vi "PH_gentec_P-Link.ProcCases.vi"(0 "i ref in":refnum<vi>, 1 "selector":string, 2 "Data":T1, 3 "call cluster":T2={"Object"="", "Selector"="", "CallType"=enum."synchronous", "Async Object"="", "Async Selector"="", "Data Descriptor"="", "Data"=[], "Error #"=0, "Expire"=0}, 5 "error in":errorcluster) -> (14 "i ref out":refnum<vi>, 17 "answer cluster":T2={"Object"="", "Selector"="", "CallType"=enum."synchronous", "Async Object"="", "Async Selector"="", "Data Descriptor"="", "Data"=[], "Error #"=0, "Expire"=0}, 19 "error out":errorcluster)   [LabVIEW 2014, in "PH_gentec_P-Link.lvlib"]
doc: "This method is called by a process from within the default case in the event loop. The methods of a class that are linked to events will be called from THIS method. Add your code here."
uses:
  PH_gentec_P-Link.lvlib
  CS_Core/CSSystem/CoreDefs/CoreDefs.call_type.ctl
  CS_Core/BaseProcess/BaseProcess.descriptor string definition.ctl
  CS_Core/CSSystem/CoreDefs/CoreDefs.rawDataType.ctl
  instr.lib/Gentec-M-Link/Driver/Type Defs/gentec-M-Link.Measurement Mode.ctl
  instr.lib/Gentec-M-Link/Driver/Type Defs/gentec-M-Link.Trigger Polarity.ctl
  instr.lib/Gentec-M-Link/Driver/Type Defs/gentec-M-Link.Trigger Source.ctl
  CS_Core/CSSystem/CoreLib/CoreLib.string 2 byte array.vi
  CS_Core/CSSystem/CoreLib/CoreLib.byte array 2 short.vi
  CS_Core/CSSystem/CoreLib/CoreLib.byte array 2 int.vi
  CS_Core/CSSystem/CoreLib/CoreLib.lvlib
  CS_Core/BaseProcess/BaseProcess.lvlib
  CS_Core/CAEObj/CAEObj.lvlib
  PH_Basics/PH_PSDBWriter/PH_PSDBWriter.lvlib
  instr.lib/Gentec-M-Link/gentec-M-Link - Driver.lvlib
  PH_Basics/PH_Powermeter_BaseClass/PH_Powermeter_BaseClass.lvlib
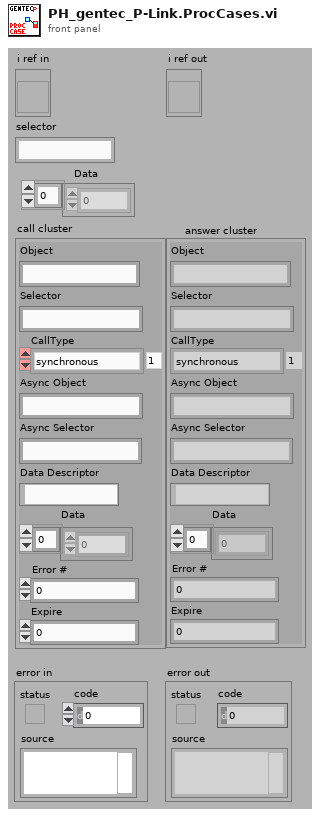
[diagram p1: front panel]
types:
  T1 = typedef "CoreDefs.rawDataType.ctl" = i8[]
  T2 = typedef "CoreDefs.call_type.ctl" = cluster{"Object":string, "Selector":string, "CallType":enum16{"simple", "synchronous", "asynchronous"}, "Async Object":string, "Async Selector":string, "Data Descriptor":T3, "Data":T1, "Error #":i32, "Expire":u32}
  T3 = typedef "BaseProcess.lvlib/BaseProcess.descriptor string definition.ctl" = string
  T4 = typedef "PH_gentec_P-Link.lvlib/PH_gentec_P-Link.i attribute.ctl" = cluster{"GUI References":cluster{"Wanted Head Settings":refnum<vi>, "Current Head Settings":refnum<vi>, "Set Auto Range":refnum<vi>, "Trigger Polarity":refnum<vi>, "Trigger Source":refnum<vi>, "Waveform Averages":refnum<vi>, "Continuous":refnum<vi>, "get one Value":refnum<vi>}, "Wanted Head Settings":T5, "Current Head Settings":T5}
  T5 = typedef "PH_gentec_P-Link.lvlib/PH_gentec_P-Link.Head Settings.ctl" = cluster{"Measurement Mode":T6, "Enable Anticipation":bool, "Set Auto Range":bool, "Block Signal":bool, "Set Head Attenuator":bool, "Enable SSE":bool, "Trigger Polarity":T7, "Trigger Source":T8, "Waveform Averages":T9, "Set Zero":i32, "Current":i32, "Start Data Flow":bool}
  T6 = typedef "gentec-M-Link - Driver.lvlib/gentec-M-Link.Measurement Mode.ctl" = u16
  T7 = typedef "gentec-M-Link - Driver.lvlib/gentec-M-Link.Trigger Polarity.ctl" = u16
  T8 = typedef "gentec-M-Link - Driver.lvlib/gentec-M-Link.Trigger Source.ctl" = u16
  T9 = typedef "gentec-M-Link - Driver.lvlib/gentec-M-Link.Waveform Averages.ctl" = u16
  T10 = typedef "PH_PSDBWriter.lvlib/PH_PSDBWriter.PHELIX-Subsystems.ctl" = i32
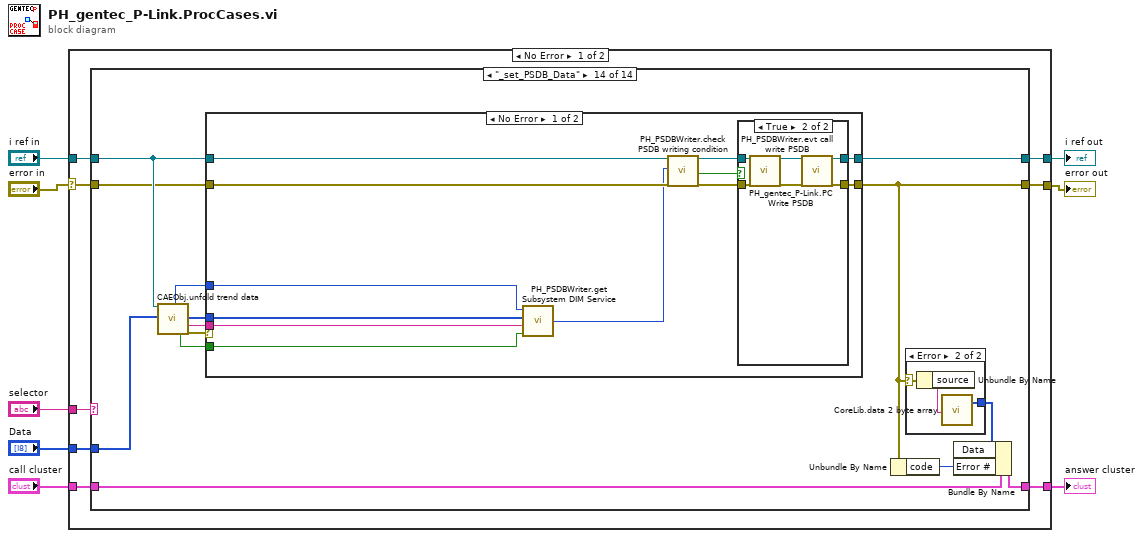
[diagram p0: block diagram]
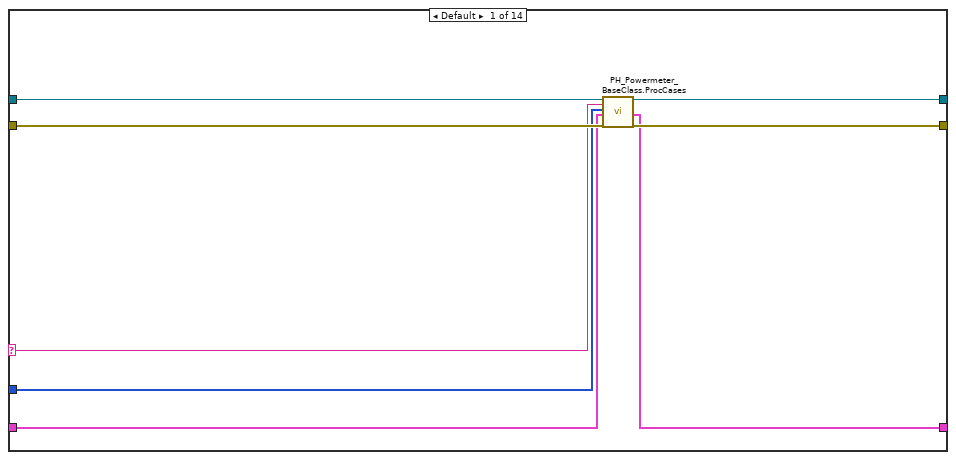
[diagram p2: hidden frame]
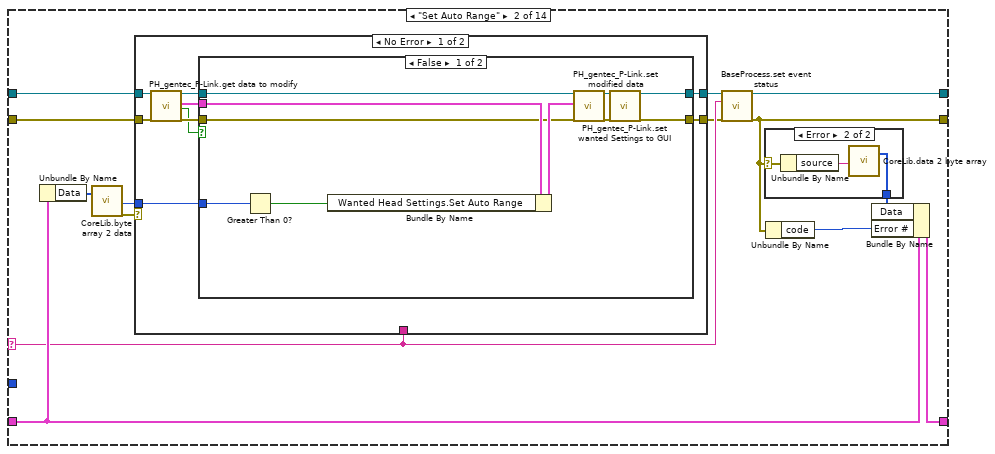
[diagram p3: hidden frame]
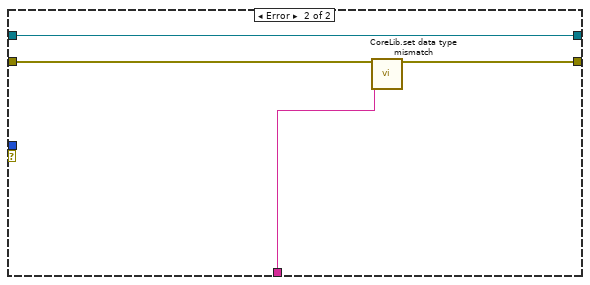
[diagram p6: hidden frame]
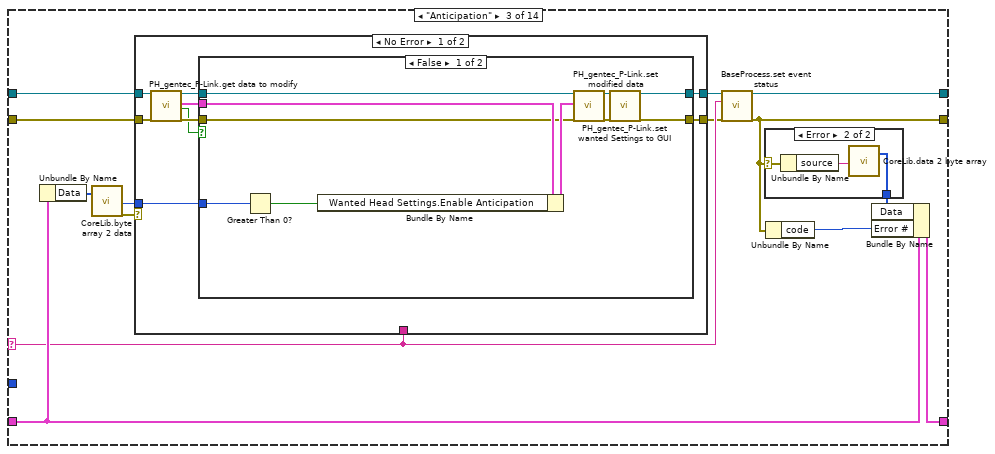
[diagram p7: hidden frame]
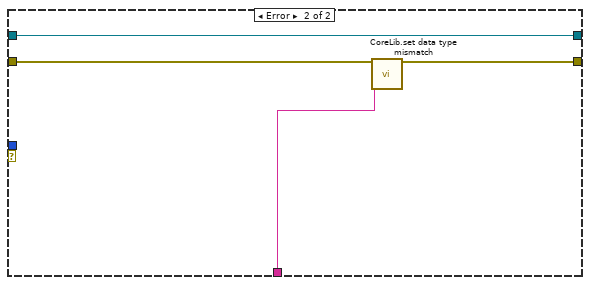
[diagram p10: hidden frame]
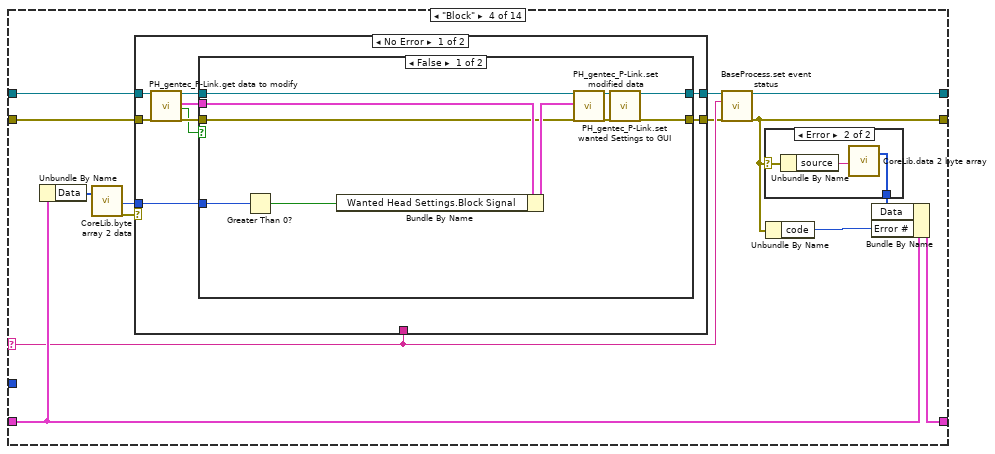
[diagram p11: hidden frame]
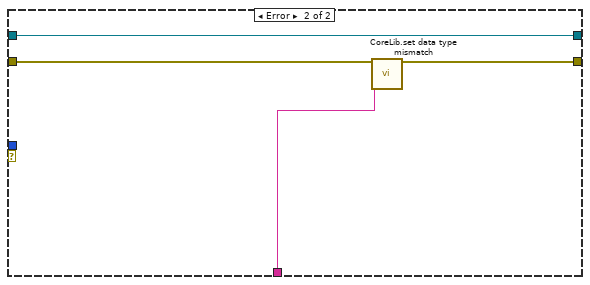
[diagram p14: hidden frame]
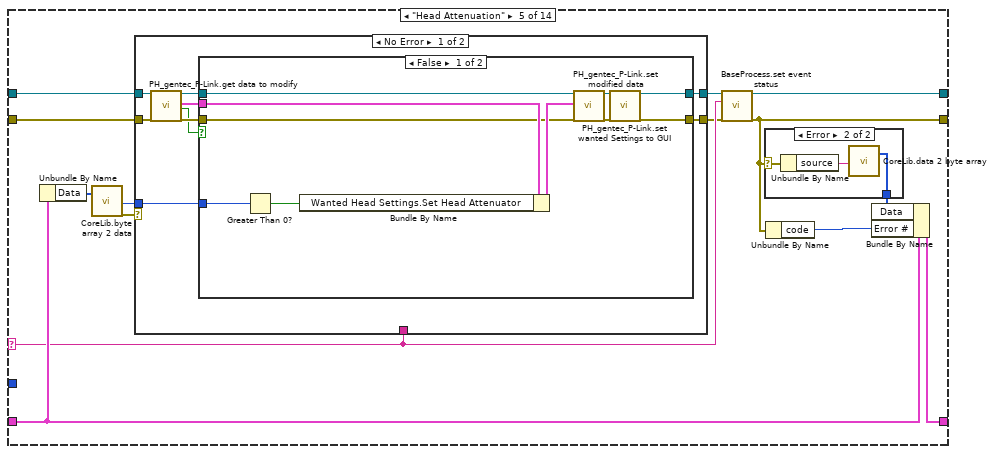
[diagram p15: hidden frame]
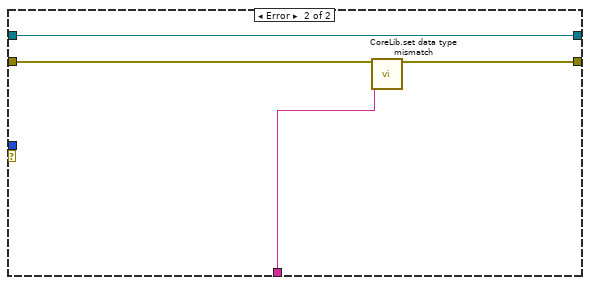
[diagram p18: hidden frame]
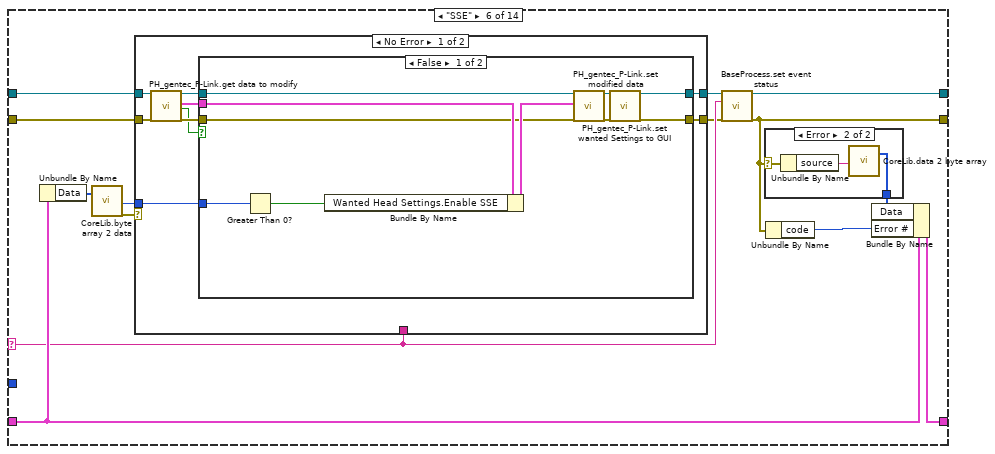
[diagram p19: hidden frame]
diagram:
  n1 = case shown="No Error" "error in" {
    selector: "error in" -> [w9 w553]
    tunnel: "selector" -> [w16 _]
    tunnel: [w15 w552] -> w7
    tunnel: "call cluster" -> [w14 w552]
    tunnel: "i ref in" -> [w13 w554]
    tunnel: [w12 w554] -> w4
    tunnel: [w11 w553] -> w1
    tunnel: "Data" -> [w10 _]
    frame No Error {
      n2 = case shown="\"_set_PSDB_Data\"" w16 {
        selector: w16 -> [w19 w32 w74 w116 w158 w200 w242 w288 w332 w376 w418 w461 w491 _]
        tunnel: w13 -> [w18 w38 w80 w122 w164 w206 w248 w294 w338 w382 w424 w467 w497 w517]
        tunnel: [w24 w33 w75 w117 w159 w201 w243 w289 w333 w377 w419 w462 w492 w516] -> w12
        tunnel: w14 -> [w20 w35 w77 w119 w161 w203 w245 w291 w335 w379 w421 w464 w494 w525]
        tunnel: [w21 w26 w68 w110 w152 w194 w236 w282 w326 w370 w412 w458 w488 w523] -> w15
        tunnel: w9 -> [w23 w37 w79 w121 w163 w205 w247 w293 w337 w381 w423 w466 w496 w514]
        tunnel: [w22 w34 w76 w118 w160 w202 w244 w290 w334 w378 w420 w463 w493 w515] -> w11
        tunnel: w10 -> [w17 _ _ _ _ _ _ _ _ _ _ _ _ w513]
        frame Default {
          # "In the default case, always call the ProcCase method of the parent class"
          n3 = call "PH_Powermeter_BaseClass.ProcCases.vi"("i ref in"=w18, "selector"=w19, "Data"=w17, "call cluster"=w20, "error in"=w23) -> ("i ref out"=w24:refnum<vi>, "answer cluster"=w21:T2, "error out"=w22:errorcluster)  [unwired: 12 in]
        }
        frame "Set Auto Range" {
          n4 = Unbundle By Name(w35) -> ("Data"=w29:T1)
          n5 = call-poly "CoreLib.byte array 2 data.vi"("byteArray"=w29) -> ("i16"=w28:i16, "error out"=w27:errorcluster)  [unwired: 16 in, 1 out]
          n6 = case shown="No Error" w27 {
            tunnel: [w48 w66] -> w30
            tunnel: w38 -> [w50 w66]
            tunnel: w37 -> [w47 w65]
            tunnel: [w45 w64] -> w31
            tunnel: w32 -> [_ w63]
            tunnel: w28 -> [w42 _]
            frame No Error {
              n7 = call "PH_gentec_P-Link.get data to modify.vi"("i ref in"=w50, "error in (no error)"=w47) -> ("i ref out"=w49:refnum<vi>, "i attribute"=w43:T4, "timed out"=w44:bool, "error out"=w46:errorcluster)  [unwired: 14 in]
              n8 = case shown="False" w44 {
                tunnel: w49 -> [w60 w62]
                tunnel: [w52 w62] -> w48
                tunnel: w46 -> [w55 w61]
                tunnel: [w51 w61] -> w45
                tunnel: w43 -> [w57 _]
                tunnel: w42 -> [w56 _]
                frame False {
                  n9 = Greater Than 0?(x=w56) -> (x > 0?=w53:bool)
                  n10 = Bundle By Name(cluster=w57, "Wanted Head Settings.Set Auto Range"=w53) -> (w58:T4)
                  n11 = call "PH_gentec_P-Link.set modified data.vi"("i ref in"=w60, "i attribute"=w58, "error in (no error)"=w55) -> ("i ref out"=w54:refnum<vi>, "error out"=w59:errorcluster)  [unwired: 15 in]
                  n12 = call "PH_gentec_P-Link.set wanted Settings to GUI.vi"("i ref in"=w54, "error in"=w59) -> ("i ref out"=w52:refnum<vi>, "error out"=w51:errorcluster)  [unwired: 16 in]
                }
                frame True {
                }
              }
            }
            frame Error {
              n13 = call "CoreLib.set data type mismatch.vi"("error in (no error)"=w65, "error source"=w63) -> ("error out"=w64:errorcluster)  [unwired: 17 in]
            }
          }
          n14 = call "BaseProcess.set event status.vi"("i ref in"=w30, "EventStatus"=w32, "error in (no error)"=w31) -> ("i ref out"=w33:refnum<vi>, "error out"=w34:errorcluster)  [unwired: 14 in, 1 out]
          n15 = case shown="Error" w34 {
            selector: w34 -> [_ w41]
            tunnel: [_ w39] -> w25
            frame No Error {
            }
            frame Error {
              n16 = Unbundle By Name(w41) -> ("source"=w40:string)
              n17 = call-poly "CoreLib.data 2 byte array.vi"("string"=w40) -> ("byteArray out"=w39:T1)  [unwired: 18 in]
            }
          }
          n18 = Unbundle By Name(w34) -> ("code"=w36:i32)
          n19 = Bundle By Name(cluster=w35, "Data"=w25, "Error #"=w36) -> (w26:T2)
        }
        frame "Anticipation" {
          n20 = Unbundle By Name(w77) -> ("Data"=w71:T1)
          n21 = call-poly "CoreLib.byte array 2 data.vi"("byteArray"=w71) -> ("i16"=w70:i16, "error out"=w69:errorcluster)  [unwired: 16 in, 1 out]
          n22 = case shown="No Error" w69 {
            tunnel: [w90 w108] -> w72
            tunnel: w80 -> [w92 w108]
            tunnel: w79 -> [w89 w107]
            tunnel: [w87 w106] -> w73
            tunnel: w74 -> [_ w105]
            tunnel: w70 -> [w84 _]
            frame No Error {
              n23 = call "PH_gentec_P-Link.get data to modify.vi"("i ref in"=w92, "error in (no error)"=w89) -> ("i ref out"=w91:refnum<vi>, "i attribute"=w85:T4, "timed out"=w86:bool, "error out"=w88:errorcluster)  [unwired: 14 in]
              n24 = case shown="False" w86 {
                tunnel: w91 -> [w102 w104]
                tunnel: [w94 w104] -> w90
                tunnel: w88 -> [w97 w103]
                tunnel: [w93 w103] -> w87
                tunnel: w85 -> [w99 _]
                tunnel: w84 -> [w98 _]
                frame False {
                  n25 = Greater Than 0?(x=w98) -> (x > 0?=w95:bool)
                  n26 = Bundle By Name(cluster=w99, "Wanted Head Settings.Enable Anticipation"=w95) -> (w100:T4)
                  n27 = call "PH_gentec_P-Link.set modified data.vi"("i ref in"=w102, "i attribute"=w100, "error in (no error)"=w97) -> ("i ref out"=w96:refnum<vi>, "error out"=w101:errorcluster)  [unwired: 15 in]
                  n28 = call "PH_gentec_P-Link.set wanted Settings to GUI.vi"("i ref in"=w96, "error in"=w101) -> ("i ref out"=w94:refnum<vi>, "error out"=w93:errorcluster)  [unwired: 16 in]
                }
                frame True {
                }
              }
            }
            frame Error {
              n29 = call "CoreLib.set data type mismatch.vi"("error in (no error)"=w107, "error source"=w105) -> ("error out"=w106:errorcluster)  [unwired: 17 in]
            }
          }
          n30 = call "BaseProcess.set event status.vi"("i ref in"=w72, "EventStatus"=w74, "error in (no error)"=w73) -> ("i ref out"=w75:refnum<vi>, "error out"=w76:errorcluster)  [unwired: 14 in, 1 out]
          n31 = case shown="Error" w76 {
            selector: w76 -> [_ w83]
            tunnel: [_ w81] -> w67
            frame No Error {
            }
            frame Error {
              n32 = Unbundle By Name(w83) -> ("source"=w82:string)
              n33 = call-poly "CoreLib.data 2 byte array.vi"("string"=w82) -> ("byteArray out"=w81:T1)  [unwired: 18 in]
            }
          }
          n34 = Unbundle By Name(w76) -> ("code"=w78:i32)
          n35 = Bundle By Name(cluster=w77, "Data"=w67, "Error #"=w78) -> (w68:T2)
        }
        frame "Block" {
          n36 = Unbundle By Name(w119) -> ("Data"=w113:T1)
          n37 = call-poly "CoreLib.byte array 2 data.vi"("byteArray"=w113) -> ("i16"=w112:i16, "error out"=w111:errorcluster)  [unwired: 16 in, 1 out]
          n38 = case shown="No Error" w111 {
            tunnel: [w132 w150] -> w114
            tunnel: w122 -> [w134 w150]
            tunnel: w121 -> [w131 w149]
            tunnel: [w129 w148] -> w115
            tunnel: w116 -> [_ w147]
            tunnel: w112 -> [w126 _]
            frame No Error {
              n39 = call "PH_gentec_P-Link.get data to modify.vi"("i ref in"=w134, "error in (no error)"=w131) -> ("i ref out"=w133:refnum<vi>, "i attribute"=w127:T4, "timed out"=w128:bool, "error out"=w130:errorcluster)  [unwired: 14 in]
              n40 = case shown="False" w128 {
                tunnel: w133 -> [w144 w146]
                tunnel: [w136 w146] -> w132
                tunnel: w130 -> [w139 w145]
                tunnel: [w135 w145] -> w129
                tunnel: w127 -> [w141 _]
                tunnel: w126 -> [w140 _]
                frame False {
                  n41 = Greater Than 0?(x=w140) -> (x > 0?=w137:bool)
                  n42 = Bundle By Name(cluster=w141, "Wanted Head Settings.Block Signal"=w137) -> (w142:T4)
                  n43 = call "PH_gentec_P-Link.set modified data.vi"("i ref in"=w144, "i attribute"=w142, "error in (no error)"=w139) -> ("i ref out"=w138:refnum<vi>, "error out"=w143:errorcluster)  [unwired: 15 in]
                  n44 = call "PH_gentec_P-Link.set wanted Settings to GUI.vi"("i ref in"=w138, "error in"=w143) -> ("i ref out"=w136:refnum<vi>, "error out"=w135:errorcluster)  [unwired: 16 in]
                }
                frame True {
                }
              }
            }
            frame Error {
              n45 = call "CoreLib.set data type mismatch.vi"("error in (no error)"=w149, "error source"=w147) -> ("error out"=w148:errorcluster)  [unwired: 17 in]
            }
          }
          n46 = call "BaseProcess.set event status.vi"("i ref in"=w114, "EventStatus"=w116, "error in (no error)"=w115) -> ("i ref out"=w117:refnum<vi>, "error out"=w118:errorcluster)  [unwired: 14 in, 1 out]
          n47 = case shown="Error" w118 {
            selector: w118 -> [_ w125]
            tunnel: [_ w123] -> w109
            frame No Error {
            }
            frame Error {
              n48 = Unbundle By Name(w125) -> ("source"=w124:string)
              n49 = call-poly "CoreLib.data 2 byte array.vi"("string"=w124) -> ("byteArray out"=w123:T1)  [unwired: 18 in]
            }
          }
          n50 = Unbundle By Name(w118) -> ("code"=w120:i32)
          n51 = Bundle By Name(cluster=w119, "Data"=w109, "Error #"=w120) -> (w110:T2)
        }
        frame "Head Attenuation" {
          n52 = Unbundle By Name(w161) -> ("Data"=w155:T1)
          n53 = call-poly "CoreLib.byte array 2 data.vi"("byteArray"=w155) -> ("i16"=w154:i16, "error out"=w153:errorcluster)  [unwired: 16 in, 1 out]
          n54 = case shown="No Error" w153 {
            tunnel: [w174 w192] -> w156
            tunnel: w164 -> [w176 w192]
            tunnel: w163 -> [w173 w191]
            tunnel: [w171 w190] -> w157
            tunnel: w158 -> [_ w189]
            tunnel: w154 -> [w168 _]
            frame No Error {
              n55 = call "PH_gentec_P-Link.get data to modify.vi"("i ref in"=w176, "error in (no error)"=w173) -> ("i ref out"=w175:refnum<vi>, "i attribute"=w169:T4, "timed out"=w170:bool, "error out"=w172:errorcluster)  [unwired: 14 in]
              n56 = case shown="False" w170 {
                tunnel: w175 -> [w186 w188]
                tunnel: [w178 w188] -> w174
                tunnel: w172 -> [w181 w187]
                tunnel: [w177 w187] -> w171
                tunnel: w169 -> [w183 _]
                tunnel: w168 -> [w182 _]
                frame False {
                  n57 = Greater Than 0?(x=w182) -> (x > 0?=w179:bool)
                  n58 = Bundle By Name(cluster=w183, "Wanted Head Settings.Set Head Attenuator"=w179) -> (w184:T4)
                  n59 = call "PH_gentec_P-Link.set modified data.vi"("i ref in"=w186, "i attribute"=w184, "error in (no error)"=w181) -> ("i ref out"=w180:refnum<vi>, "error out"=w185:errorcluster)  [unwired: 15 in]
                  n60 = call "PH_gentec_P-Link.set wanted Settings to GUI.vi"("i ref in"=w180, "error in"=w185) -> ("i ref out"=w178:refnum<vi>, "error out"=w177:errorcluster)  [unwired: 16 in]
                }
                frame True {
                }
              }
            }
            frame Error {
              n61 = call "CoreLib.set data type mismatch.vi"("error in (no error)"=w191, "error source"=w189) -> ("error out"=w190:errorcluster)  [unwired: 17 in]
            }
          }
          n62 = call "BaseProcess.set event status.vi"("i ref in"=w156, "EventStatus"=w158, "error in (no error)"=w157) -> ("i ref out"=w159:refnum<vi>, "error out"=w160:errorcluster)  [unwired: 14 in, 1 out]
          n63 = case shown="Error" w160 {
            selector: w160 -> [_ w167]
            tunnel: [_ w165] -> w151
            frame No Error {
            }
            frame Error {
              n64 = Unbundle By Name(w167) -> ("source"=w166:string)
              n65 = call-poly "CoreLib.data 2 byte array.vi"("string"=w166) -> ("byteArray out"=w165:T1)  [unwired: 18 in]
            }
          }
          n66 = Unbundle By Name(w160) -> ("code"=w162:i32)
          n67 = Bundle By Name(cluster=w161, "Data"=w151, "Error #"=w162) -> (w152:T2)
        }
        frame "SSE" {
          n68 = Unbundle By Name(w203) -> ("Data"=w197:T1)
          n69 = call-poly "CoreLib.byte array 2 data.vi"("byteArray"=w197) -> ("i16"=w196:i16, "error out"=w195:errorcluster)  [unwired: 16 in, 1 out]
          n70 = case shown="No Error" w195 {
            tunnel: [w216 w234] -> w198
            tunnel: w206 -> [w218 w234]
            tunnel: w205 -> [w215 w233]
            tunnel: [w213 w232] -> w199
            tunnel: w200 -> [_ w231]
            tunnel: w196 -> [w210 _]
            frame No Error {
              n71 = call "PH_gentec_P-Link.get data to modify.vi"("i ref in"=w218, "error in (no error)"=w215) -> ("i ref out"=w217:refnum<vi>, "i attribute"=w211:T4, "timed out"=w212:bool, "error out"=w214:errorcluster)  [unwired: 14 in]
              n72 = case shown="False" w212 {
                tunnel: w217 -> [w228 w230]
                tunnel: [w220 w230] -> w216
                tunnel: w214 -> [w223 w229]
                tunnel: [w219 w229] -> w213
                tunnel: w211 -> [w225 _]
                tunnel: w210 -> [w224 _]
                frame False {
                  n73 = Greater Than 0?(x=w224) -> (x > 0?=w221:bool)
                  n74 = Bundle By Name(cluster=w225, "Wanted Head Settings.Enable SSE"=w221) -> (w226:T4)
                  n75 = call "PH_gentec_P-Link.set modified data.vi"("i ref in"=w228, "i attribute"=w226, "error in (no error)"=w223) -> ("i ref out"=w222:refnum<vi>, "error out"=w227:errorcluster)  [unwired: 15 in]
                  n76 = call "PH_gentec_P-Link.set wanted Settings to GUI.vi"("i ref in"=w222, "error in"=w227) -> ("i ref out"=w220:refnum<vi>, "error out"=w219:errorcluster)  [unwired: 16 in]
                }
                frame True {
                }
              }
            }
            frame Error {
              n77 = call "CoreLib.set data type mismatch.vi"("error in (no error)"=w233, "error source"=w231) -> ("error out"=w232:errorcluster)  [unwired: 17 in]
            }
          }
          n78 = call "BaseProcess.set event status.vi"("i ref in"=w198, "EventStatus"=w200, "error in (no error)"=w199) -> ("i ref out"=w201:refnum<vi>, "error out"=w202:errorcluster)  [unwired: 14 in, 1 out]
          n79 = case shown="Error" w202 {
            selector: w202 -> [_ w209]
            tunnel: [_ w207] -> w193
            frame No Error {
            }
            frame Error {
              n80 = Unbundle By Name(w209) -> ("source"=w208:string)
              n81 = call-poly "CoreLib.data 2 byte array.vi"("string"=w208) -> ("byteArray out"=w207:T1)  [unwired: 18 in]
            }
          }
          n82 = Unbundle By Name(w202) -> ("code"=w204:i32)
          n83 = Bundle By Name(cluster=w203, "Data"=w193, "Error #"=w204) -> (w194:T2)
        }
        frame "Measurement Mode" {
          n84 = Unbundle By Name(w245) -> ("Data"=w239:T1)
          n85 = call-poly "CoreLib.byte array 2 data.vi"("byteArray"=w239) -> ("i32"=w238:i32, "error out"=w237:errorcluster)  [unwired: 16 in, 1 out]
          n86 = case shown="No Error" w237 {
            tunnel: [w258 w280] -> w240
            tunnel: w248 -> [w260 w280]
            tunnel: w247 -> [w257 w279]
            tunnel: [w255 w278] -> w241
            tunnel: w242 -> [_ w277]
            tunnel: w238 -> [w252 _]
            frame No Error {
              n87 = call "PH_gentec_P-Link.get data to modify.vi"("i ref in"=w260, "error in (no error)"=w257) -> ("i ref out"=w259:refnum<vi>, "i attribute"=w253:T4, "timed out"=w254:bool, "error out"=w256:errorcluster)  [unwired: 14 in]
              n88 = case shown="False" w254 {
                tunnel: w259 -> [w274 w276]
                tunnel: [w262 w276] -> w258
                tunnel: w256 -> [w271 w275]
                tunnel: [w261 w275] -> w255
                tunnel: w253 -> [w269 _]
                tunnel: w252 -> [w268 _]
                frame False {
                  w264 = T6 1 items=["other Mode", "Energymode"] ("Wanted Head Settings.Measurement Mode")
                  w265 = T6 0 items=["other Mode", "Energymode"] ("Wanted Head Settings.Measurement Mode")
                  n89 = Equal?(x=w268, y=1) -> (x = y?=w266:bool)
                  n90 = Select(t=w264, s=w266, f=w265) -> (s? t:f=w263:T6)
                  n91 = Bundle By Name(cluster=w269, "Wanted Head Settings.Measurement Mode"=w263) -> (w272:T4)
                  n92 = call "PH_gentec_P-Link.set modified data.vi"("i ref in"=w274, "i attribute"=w272, "error in (no error)"=w271) -> ("i ref out"=w270:refnum<vi>, "error out"=w273:errorcluster)  [unwired: 15 in]
                  n93 = call "PH_gentec_P-Link.set wanted Settings to GUI.vi"("i ref in"=w270, "error in"=w273) -> ("i ref out"=w262:refnum<vi>, "error out"=w261:errorcluster)  [unwired: 16 in]
                }
                frame True {
                }
              }
            }
            frame Error {
              n94 = call "CoreLib.set data type mismatch.vi"("error in (no error)"=w279, "error source"=w277) -> ("error out"=w278:errorcluster)  [unwired: 17 in]
            }
          }
          n95 = call "BaseProcess.set event status.vi"("i ref in"=w240, "EventStatus"=w242, "error in (no error)"=w241) -> ("i ref out"=w243:refnum<vi>, "error out"=w244:errorcluster)  [unwired: 14 in, 1 out]
          n96 = case shown="Error" w244 {
            selector: w244 -> [_ w251]
            tunnel: [_ w249] -> w235
            frame No Error {
            }
            frame Error {
              n97 = Unbundle By Name(w251) -> ("source"=w250:string)
              n98 = call-poly "CoreLib.data 2 byte array.vi"("string"=w250) -> ("byteArray out"=w249:T1)  [unwired: 18 in]
            }
          }
          n99 = Unbundle By Name(w244) -> ("code"=w246:i32)
          n100 = Bundle By Name(cluster=w245, "Data"=w235, "Error #"=w246) -> (w236:T2)
        }
        frame "Set Trigger Polarity" {
          n101 = Unbundle By Name(w291) -> ("Data"=w285:T1)
          n102 = call-poly "CoreLib.byte array 2 data.vi"("byteArray"=w285) -> ("i32"=w284:i32, "error out"=w283:errorcluster)  [unwired: 16 in, 1 out]
          n103 = case shown="No Error" w283 {
            tunnel: [w304 w324] -> w286
            tunnel: w294 -> [w306 w324]
            tunnel: w293 -> [w303 w323]
            tunnel: [w301 w322] -> w287
            tunnel: w288 -> [_ w321]
            tunnel: w284 -> [w298 _]
            frame No Error {
              n104 = call "PH_gentec_P-Link.get data to modify.vi"("i ref in"=w306, "error in (no error)"=w303) -> ("i ref out"=w305:refnum<vi>, "i attribute"=w299:T4, "timed out"=w300:bool, "error out"=w302:errorcluster)  [unwired: 14 in]
              n105 = case shown="False" w300 {
                tunnel: w305 -> [w316 w320]
                tunnel: [w308 w320] -> w304
                tunnel: w302 -> [w313 w319]
                tunnel: [w307 w319] -> w301
                tunnel: w299 -> [w311 _]
                tunnel: w298 -> [w309 _]
                frame False {
                  n106 = case shown="Default" w309 {
                    tunnel: [w317 w318] -> w310
                    frame 1 {
                      w317 = T7 1 items=["Rising Edge", "Falling Edge"] ("Wanted Head Settings.Trigger Polarity")
                    }
                    frame Default {
                      w318 = T7 0 items=["Rising Edge", "Falling Edge"] ("Wanted Head Settings.Trigger Polarity")
                    }
                  }
                  n107 = Bundle By Name(cluster=w311, "Wanted Head Settings.Trigger Polarity"=w310) -> (w314:T4)
                  n108 = call "PH_gentec_P-Link.set modified data.vi"("i ref in"=w316, "i attribute"=w314, "error in (no error)"=w313) -> ("i ref out"=w312:refnum<vi>, "error out"=w315:errorcluster)  [unwired: 15 in]
                  n109 = call "PH_gentec_P-Link.set wanted Settings to GUI.vi"("i ref in"=w312, "error in"=w315) -> ("i ref out"=w308:refnum<vi>, "error out"=w307:errorcluster)  [unwired: 16 in]
                }
                frame True {
                }
              }
            }
            frame Error {
              n110 = call "CoreLib.set data type mismatch.vi"("error in (no error)"=w323, "error source"=w321) -> ("error out"=w322:errorcluster)  [unwired: 17 in]
            }
          }
          n111 = call "BaseProcess.set event status.vi"("i ref in"=w286, "EventStatus"=w288, "error in (no error)"=w287) -> ("i ref out"=w289:refnum<vi>, "error out"=w290:errorcluster)  [unwired: 14 in, 1 out]
          n112 = case shown="Error" w290 {
            selector: w290 -> [_ w297]
            tunnel: [_ w295] -> w281
            frame No Error {
            }
            frame Error {
              n113 = Unbundle By Name(w297) -> ("source"=w296:string)
              n114 = call-poly "CoreLib.data 2 byte array.vi"("string"=w296) -> ("byteArray out"=w295:T1)  [unwired: 18 in]
            }
          }
          n115 = Unbundle By Name(w290) -> ("code"=w292:i32)
          n116 = Bundle By Name(cluster=w291, "Data"=w281, "Error #"=w292) -> (w282:T2)
        }
        frame "Set Trigger Source" {
          n117 = Unbundle By Name(w335) -> ("Data"=w329:T1)
          n118 = call-poly "CoreLib.byte array 2 data.vi"("byteArray"=w329) -> ("i32"=w328:i32, "error out"=w327:errorcluster)  [unwired: 16 in, 1 out]
          n119 = case shown="No Error" w327 {
            tunnel: [w348 w368] -> w330
            tunnel: w338 -> [w350 w368]
            tunnel: w337 -> [w347 w367]
            tunnel: [w345 w366] -> w331
            tunnel: w332 -> [_ w365]
            tunnel: w328 -> [w342 _]
            frame No Error {
              n120 = call "PH_gentec_P-Link.get data to modify.vi"("i ref in"=w350, "error in (no error)"=w347) -> ("i ref out"=w349:refnum<vi>, "i attribute"=w343:T4, "timed out"=w344:bool, "error out"=w346:errorcluster)  [unwired: 14 in]
              n121 = case shown="False" w344 {
                tunnel: w349 -> [w360 w364]
                tunnel: [w352 w364] -> w348
                tunnel: w346 -> [w357 w363]
                tunnel: [w351 w363] -> w345
                tunnel: w343 -> [w355 _]
                tunnel: w342 -> [w354 _]
                frame False {
                  n122 = case shown="0" w354 {
                    tunnel: [w361 w362] -> w353
                    frame 0 {
                      w361 = T8 0 items=["Internal", "External"] ("Wanted Head Settings.Trigger Source")
                    }
                    frame Default {
                      w362 = T8 1 items=["Internal", "External"] ("Wanted Head Settings.Trigger Source")
                    }
                  }
                  n123 = Bundle By Name(cluster=w355, "Wanted Head Settings.Trigger Source"=w353) -> (w358:T4)
                  n124 = call "PH_gentec_P-Link.set modified data.vi"("i ref in"=w360, "i attribute"=w358, "error in (no error)"=w357) -> ("i ref out"=w356:refnum<vi>, "error out"=w359:errorcluster)  [unwired: 15 in]
                  n125 = call "PH_gentec_P-Link.set wanted Settings to GUI.vi"("i ref in"=w356, "error in"=w359) -> ("i ref out"=w352:refnum<vi>, "error out"=w351:errorcluster)  [unwired: 16 in]
                }
                frame True {
                }
              }
            }
            frame Error {
              n126 = call "CoreLib.set data type mismatch.vi"("error in (no error)"=w367, "error source"=w365) -> ("error out"=w366:errorcluster)  [unwired: 17 in]
            }
          }
          n127 = call "BaseProcess.set event status.vi"("i ref in"=w330, "EventStatus"=w332, "error in (no error)"=w331) -> ("i ref out"=w333:refnum<vi>, "error out"=w334:errorcluster)  [unwired: 14 in, 1 out]
          n128 = case shown="Error" w334 {
            selector: w334 -> [_ w341]
            tunnel: [_ w339] -> w325
            frame No Error {
            }
            frame Error {
              n129 = Unbundle By Name(w341) -> ("source"=w340:string)
              n130 = call-poly "CoreLib.data 2 byte array.vi"("string"=w340) -> ("byteArray out"=w339:T1)  [unwired: 18 in]
            }
          }
          n131 = Unbundle By Name(w334) -> ("code"=w336:i32)
          n132 = Bundle By Name(cluster=w335, "Data"=w325, "Error #"=w336) -> (w326:T2)
        }
        frame "Set Waveform Averages" {
          n133 = Unbundle By Name(w379) -> ("Data"=w373:T1)
          n134 = call-poly "CoreLib.byte array 2 data.vi"("byteArray"=w373) -> ("i32"=w372:i32, "error out"=w371:errorcluster)  [unwired: 16 in, 1 out]
          n135 = case shown="No Error" w371 {
            tunnel: [w392 w410] -> w374
            tunnel: w382 -> [w394 w410]
            tunnel: w381 -> [w391 w409]
            tunnel: [w389 w408] -> w375
            tunnel: w376 -> [_ w407]
            tunnel: w372 -> [w386 _]
            frame No Error {
              n136 = call "PH_gentec_P-Link.get data to modify.vi"("i ref in"=w394, "error in (no error)"=w391) -> ("i ref out"=w393:refnum<vi>, "i attribute"=w387:T4, "timed out"=w388:bool, "error out"=w390:errorcluster)  [unwired: 14 in]
              n137 = case shown="False" w388 {
                tunnel: w393 -> [w404 w406]
                tunnel: [w396 w406] -> w392
                tunnel: w390 -> [w401 w405]
                tunnel: [w395 w405] -> w389
                tunnel: w387 -> [w399 _]
                tunnel: w386 -> [w398 _]
                frame False {
                  n138 = To Unsigned Word Integer(number=w398) -> (unsigned 16bit integer=w397:u16)
                  n139 = Bundle By Name(cluster=w399, "Wanted Head Settings.Waveform Averages"=w397) -> (w402:T4)
                  n140 = call "PH_gentec_P-Link.set modified data.vi"("i ref in"=w404, "i attribute"=w402, "error in (no error)"=w401) -> ("i ref out"=w400:refnum<vi>, "error out"=w403:errorcluster)  [unwired: 15 in]
                  n141 = call "PH_gentec_P-Link.set wanted Settings to GUI.vi"("i ref in"=w400, "error in"=w403) -> ("i ref out"=w396:refnum<vi>, "error out"=w395:errorcluster)  [unwired: 16 in]
                }
                frame True {
                }
              }
            }
            frame Error {
              n142 = call "CoreLib.set data type mismatch.vi"("error in (no error)"=w409, "error source"=w407) -> ("error out"=w408:errorcluster)  [unwired: 17 in]
            }
          }
          n143 = call "BaseProcess.set event status.vi"("i ref in"=w374, "EventStatus"=w376, "error in (no error)"=w375) -> ("i ref out"=w377:refnum<vi>, "error out"=w378:errorcluster)  [unwired: 14 in, 1 out]
          n144 = case shown="Error" w378 {
            selector: w378 -> [_ w385]
            tunnel: [_ w383] -> w369
            frame No Error {
            }
            frame Error {
              n145 = Unbundle By Name(w385) -> ("source"=w384:string)
              n146 = call-poly "CoreLib.data 2 byte array.vi"("string"=w384) -> ("byteArray out"=w383:T1)  [unwired: 18 in]
            }
          }
          n147 = Unbundle By Name(w378) -> ("code"=w380:i32)
          n148 = Bundle By Name(cluster=w379, "Data"=w369, "Error #"=w380) -> (w370:T2)
        }
        frame "Continuous Measurement" {
          n149 = Unbundle By Name(w421) -> ("Data"=w415:T1)
          n150 = call-poly "CoreLib.byte array 2 data.vi"("byteArray"=w415) -> ("i16"=w414:i16, "error out"=w413:errorcluster)  [unwired: 16 in, 1 out]
          n151 = case shown="No Error" w413 {
            tunnel: [w434 w452] -> w416
            tunnel: w424 -> [w436 w452]
            tunnel: w423 -> [w433 w451]
            tunnel: [w431 w450] -> w417
            tunnel: w418 -> [_ w449]
            tunnel: w414 -> [w428 _]
            frame No Error {
              n152 = call "PH_gentec_P-Link.get data to modify.vi"("i ref in"=w436, "error in (no error)"=w433) -> ("i ref out"=w435:refnum<vi>, "i attribute"=w429:T4, "timed out"=w430:bool, "error out"=w432:errorcluster)  [unwired: 14 in]
              n153 = case shown="False" w430 {
                tunnel: w435 -> [w446 w448]
                tunnel: [w438 w448] -> w434
                tunnel: w432 -> [w441 w447]
                tunnel: [w437 w447] -> w431
                tunnel: w429 -> [w443 _]
                tunnel: w428 -> [w442 _]
                frame False {
                  n154 = Greater Than 0?(x=w442) -> (x > 0?=w439:bool)
                  n155 = Bundle By Name(cluster=w443, "Wanted Head Settings.Start Data Flow"=w439) -> (w444:T4)
                  n156 = call "PH_gentec_P-Link.set modified data.vi"("i ref in"=w446, "i attribute"=w444, "error in (no error)"=w441) -> ("i ref out"=w440:refnum<vi>, "error out"=w445:errorcluster)  [unwired: 15 in]
                  n157 = call "PH_gentec_P-Link.set wanted Settings to GUI.vi"("i ref in"=w440, "error in"=w445) -> ("i ref out"=w438:refnum<vi>, "error out"=w437:errorcluster)  [unwired: 16 in]
                }
                frame True {
                }
              }
            }
            frame Error {
              n158 = call "CoreLib.set data type mismatch.vi"("error in (no error)"=w451, "error source"=w449) -> ("error out"=w450:errorcluster)  [unwired: 17 in]
            }
          }
          n159 = call "BaseProcess.set event status.vi"("i ref in"=w416, "EventStatus"=w418, "error in (no error)"=w417) -> ("i ref out"=w419:refnum<vi>, "error out"=w420:errorcluster)  [unwired: 14 in, 1 out]
          n160 = case shown="Error" w420 {
            selector: w420 -> [_ w427]
            tunnel: [_ w425] -> w411
            frame No Error {
            }
            frame Error {
              n161 = Unbundle By Name(w427) -> ("source"=w426:string)
              n162 = call-poly "CoreLib.data 2 byte array.vi"("string"=w426) -> ("byteArray out"=w425:T1)  [unwired: 18 in]
            }
          }
          n163 = Unbundle By Name(w420) -> ("code"=w422:i32)
          n164 = Bundle By Name(cluster=w421, "Data"=w411, "Error #"=w422) -> (w412:T2)
        }
        frame "Current Measurement" {
          n165 = call "PH_gentec_P-Link.get data to modify.vi"("i ref in"=w467, "error in (no error)"=w466) -> ("i ref out"=w456:refnum<vi>, "i attribute"=w453:T4, "timed out"=w454:bool, "error out"=w455:errorcluster)  [unwired: 14 in]
          n166 = case shown="False" w454 {
            tunnel: w456 -> [w477 w479]
            tunnel: [w469 w479] -> w459
            tunnel: w455 -> [w474 w478]
            tunnel: [w468 w478] -> w460
            tunnel: w453 -> [w472 _]
            frame False {
              n167 = Unbundle By Name(w472) -> ("Wanted Head Settings.Current"=w471:i32)
              n168 = Increment(x=w471) -> (x+1=w470:i32)
              n169 = Bundle By Name(cluster=w472, "Wanted Head Settings.Current"=w470) -> (w475:T4)
              n170 = call "PH_gentec_P-Link.set modified data.vi"("i ref in"=w477, "i attribute"=w475, "error in (no error)"=w474) -> ("i ref out"=w473:refnum<vi>, "error out"=w476:errorcluster)  [unwired: 15 in]
              n171 = call "PH_gentec_P-Link.set wanted Settings to GUI.vi"("i ref in"=w473, "error in"=w476) -> ("i ref out"=w469:refnum<vi>, "error out"=w468:errorcluster)  [unwired: 16 in]
            }
            frame True {
            }
          }
          n172 = call "BaseProcess.set event status.vi"("i ref in"=w459, "EventStatus"=w461, "error in (no error)"=w460) -> ("i ref out"=w462:refnum<vi>, "error out"=w463:errorcluster)  [unwired: 14 in, 1 out]
          n173 = case shown="Error" w463 {
            selector: w463 -> [_ w482]
            tunnel: [_ w480] -> w457
            frame No Error {
            }
            frame Error {
              n174 = Unbundle By Name(w482) -> ("source"=w481:string)
              n175 = call-poly "CoreLib.data 2 byte array.vi"("string"=w481) -> ("byteArray out"=w480:T1)  [unwired: 18 in]
            }
          }
          n176 = Unbundle By Name(w463) -> ("code"=w465:i32)
          n177 = Bundle By Name(cluster=w464, "Data"=w457, "Error #"=w465) -> (w458:T2)
        }
        frame "Zero" {
          n178 = call "PH_gentec_P-Link.get data to modify.vi"("i ref in"=w497, "error in (no error)"=w496) -> ("i ref out"=w486:refnum<vi>, "i attribute"=w483:T4, "timed out"=w484:bool, "error out"=w485:errorcluster)  [unwired: 14 in]
          n179 = case shown="False" w484 {
            tunnel: w486 -> [w507 w509]
            tunnel: [w499 w509] -> w489
            tunnel: w485 -> [w504 w508]
            tunnel: [w498 w508] -> w490
            tunnel: w483 -> [w502 _]
            frame False {
              n180 = Unbundle By Name(w502) -> ("Wanted Head Settings.Set Zero"=w501:i32)
              n181 = Increment(x=w501) -> (x+1=w500:i32)
              n182 = Bundle By Name(cluster=w502, "Wanted Head Settings.Set Zero"=w500) -> (w505:T4)
              n183 = call "PH_gentec_P-Link.set modified data.vi"("i ref in"=w507, "i attribute"=w505, "error in (no error)"=w504) -> ("i ref out"=w503:refnum<vi>, "error out"=w506:errorcluster)  [unwired: 15 in]
              n184 = call "PH_gentec_P-Link.set wanted Settings to GUI.vi"("i ref in"=w503, "error in"=w506) -> ("i ref out"=w499:refnum<vi>, "error out"=w498:errorcluster)  [unwired: 16 in]
            }
            frame True {
            }
          }
          n185 = call "BaseProcess.set event status.vi"("i ref in"=w489, "EventStatus"=w491, "error in (no error)"=w490) -> ("i ref out"=w492:refnum<vi>, "error out"=w493:errorcluster)  [unwired: 14 in, 1 out]
          n186 = case shown="Error" w493 {
            selector: w493 -> [_ w512]
            tunnel: [_ w510] -> w487
            frame No Error {
            }
            frame Error {
              n187 = Unbundle By Name(w512) -> ("source"=w511:string)
              n188 = call-poly "CoreLib.data 2 byte array.vi"("string"=w511) -> ("byteArray out"=w510:T1)  [unwired: 18 in]
            }
          }
          n189 = Unbundle By Name(w493) -> ("code"=w495:i32)
          n190 = Bundle By Name(cluster=w494, "Data"=w487, "Error #"=w495) -> (w488:T2)
        }
        frame "_set_PSDB_Data" {
          n191 = call "CAEObj.unfold trend data.vi"("i ref in"=w517, "raw trend data"=w513) -> ("quality"=w522:i32, "no link"=w519:bool, "data"=w521:i8[], "typeDescriptor"=w520:string, "error out"=w518:errorcluster)  [unwired: 9 in, 4 out]
          n192 = case shown="No Error" w518 {
            tunnel: w514 -> [w538 w548]
            tunnel: [w537 w547] -> w516
            tunnel: [w536 w548] -> w515
            tunnel: w517 -> [w534 w547]
            tunnel: w519 -> [w527 _]
            tunnel: w520 -> [w529 _]
            tunnel: w521 -> [w530 _]
            tunnel: w522 -> [w528 _]
            frame No Error {
              n193 = call "PH_PSDBWriter.get Subsystem DIM Service.vi"("no link"=w527, "typeDescriptor"=w529, "data"=w530, "quality"=w528) -> ("PHELIX Subsystems"=w531:T10)
              n194 = call "PH_PSDBWriter.check PSDB writing condition.vi"("i ref in"=w534, "wanted Subsystem"=w531, "error IO"=w538) -> ("i ref out"=w533:refnum<vi>, "write PSDB?"=w532:bool, "error out"=w535:errorcluster)  [unwired: 14 in]
              n195 = case shown="True" w532 {
                tunnel: w535 -> [w539 w546]
                tunnel: [w540 w543] -> w537
                tunnel: [w539 w541] -> w536
                tunnel: w533 -> [w540 w545]
                frame False {
                }
                frame True {
                  n196 = call "PH_gentec_P-Link.PC Write PSDB.vi"("i ref in"=w545, "error IO"=w546) -> ("i ref out"=w544:refnum<vi>, "error out"=w542:errorcluster)  [unwired: 16 in]
                  n197 = call "PH_PSDBWriter.evt call write PSDB.vi"("i ref in"=w544, "error in (no error)"=w542) -> ("i ref out"=w543:refnum<vi>, "error out"=w541:errorcluster)  [unwired: 16 in]
                }
              }
            }
            frame Error {
            }
          }
          n198 = Unbundle By Name(w515) -> ("code"=w526:i32)
          n199 = case shown="Error" w515 {
            selector: w515 -> [_ w551]
            tunnel: [_ w549] -> w524
            frame No Error {
              (unwired) ""
            }
            frame Error {
              n200 = Unbundle By Name(w551) -> ("source"=w550:string)
              n201 = call-poly "CoreLib.data 2 byte array.vi"("string"=w550) -> ("byteArray out"=w549:T1)  [unwired: 18 in]
            }
          }
          n202 = Bundle By Name(cluster=w525, "Data"=w524, "Error #"=w526) -> (w523:T2)
        }
      }
    }
    frame Error {
    }
  }
  "answer cluster" <- w7
  "i ref out" <- w4
  "error out" <- w1
